vi "Current Range.vi"(8 "error in (no error)":errorcluster, 9 "Current range":T1(ring), 11 "Reference in":T2={"Device"="GPIB0::4::INSTR", "Function"="", "delay"=20, "Resolution"=0}) -> (0 "error out":errorcluster, 3 "Reference out":T2={"Device"="GPIB0::4::INSTR", "Function"="", "delay"=20, "Resolution"=0}, 4 "question out":string)   [LabVIEW 2021, in "Rigol DM3052.lvlib"]
uses:
  Rigol DM3052.lvlib
  Reference.ctl
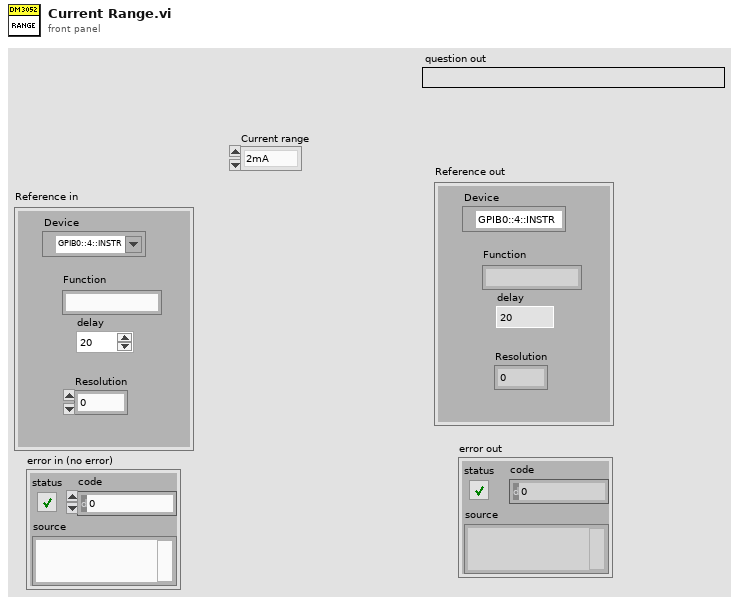
[diagram p1: front panel]
types:
  T1 = enum16{"2mA", "20mA", "200mA", "1A", "10A", "Auto"}
  T2 = typedef "Rigol DM3052.lvlib/Reference.ctl" = cluster{"Device":refnum<visa-resource-name>, "Function":string, "delay":u32, "Resolution":i8}
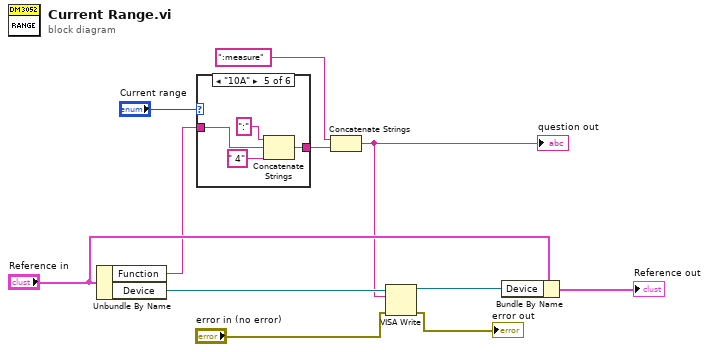
[diagram p0: block diagram]
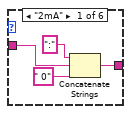
[diagram p2: hidden frame]
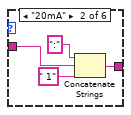
[diagram p3: hidden frame]
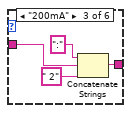
[diagram p4: hidden frame]
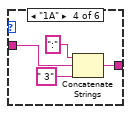
[diagram p5: hidden frame]
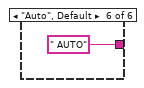
[diagram p6: hidden frame]
diagram:
  n1 = Unbundle By Name("Reference in") -> ("Function"=w4:string, "Device"=w6:refnum<visa-resource-name>)
  n2 = case shown="\"10A\"" "Current range" {
    tunnel: w4 -> [w14 w16 w20 w24 w28 _]
    tunnel: [w15 w17 w21 w25 w29 " AUTO"] -> w3
    frame "2mA" {
      n3 = Concatenate Strings(":" ("string"), w14, " 0" ("string")) -> (w15:string)
    }
    frame "20mA" {
      n4 = Concatenate Strings(":" ("string"), w16, " 1" ("string")) -> (w17:string)
    }
    frame "200mA" {
      n5 = Concatenate Strings(":" ("string"), w20, " 2" ("string")) -> (w21:string)
    }
    frame "1A" {
      n6 = Concatenate Strings(":" ("string"), w24, " 3" ("string")) -> (w25:string)
    }
    frame "10A" {
      n7 = Concatenate Strings(":" ("string"), w28, " 4" ("string")) -> (w29:string)
    }
    frame "Auto", Default {
    }
  }
  n8 = Concatenate Strings(":measure", w3) -> (w1:string)
  "question out" <- w1
  n9 = VISA Write(VISA resource name=w6, write buffer=w1, error in (no error)="error in (no error)") -> (VISA resource name out=w8:refnum<visa-resource-name>, error out=→"error out":errorcluster)  [unwired: 1 out]
  n10 = Bundle By Name(cluster="Reference in", "Device"=w8) -> (→"Reference out":T2)
